vi "main.vi"() -> ()   [LabVIEW 2023]
uses:
  GlobalVariable/SystemMotionLogic.ctl
  Vls/GlobalVariant.vi
  <vilib>/Instr/_visa.llb/VISA Configure Serial Port (Instr).vi
panel:
  in  "Numeric":i32
  in  "StrList":i32[](listbox)
  in  "HexSend":bool
  in  "ClearScreen":bool
  in  "HexDis":bool
  in  "TerminationChar":u8=10 format="%x"
  out "BuffPanel":string
  in  "SendBuffer":string
  in  "BlankButton":bool
  out "IgnoreError":errorcluster
  out "ReadBuffer":string
  in  "Error":errorcluster
  in  "BaudRate":u32=9600
  in  "VISAName":refnum<visa-resource-name>
  in  "Open":bool
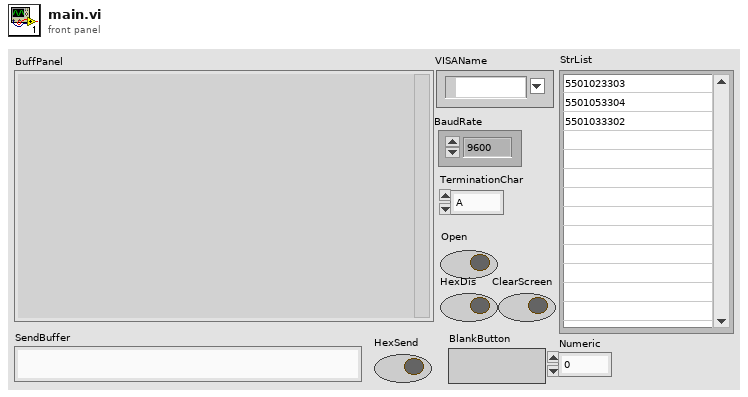
[diagram p1: front panel]
types:
  T1 = typedef "SystemMotionLogic.ctl" = enum16{"VariantInit", "FunctInit", "IdleState"}
  T2 = typedef "LVPoint32TypeDef.ctl" = cluster{"Horizontal":i32, "Vertical":i32}
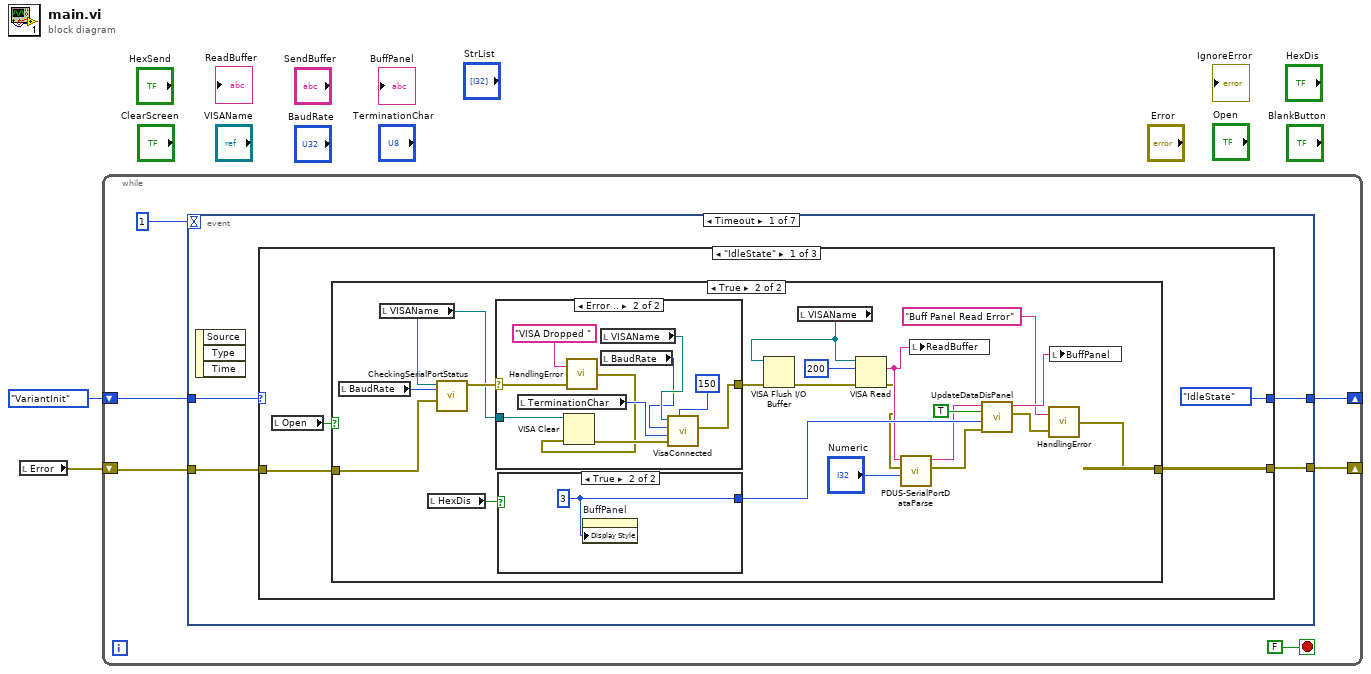
[diagram p0: block diagram]
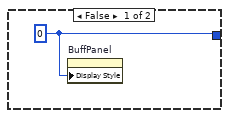
[diagram p4: hidden frame]
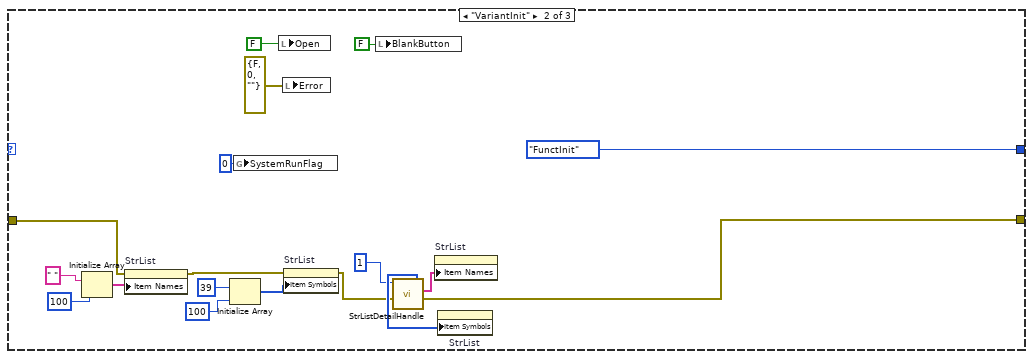
[diagram p5: hidden frame]
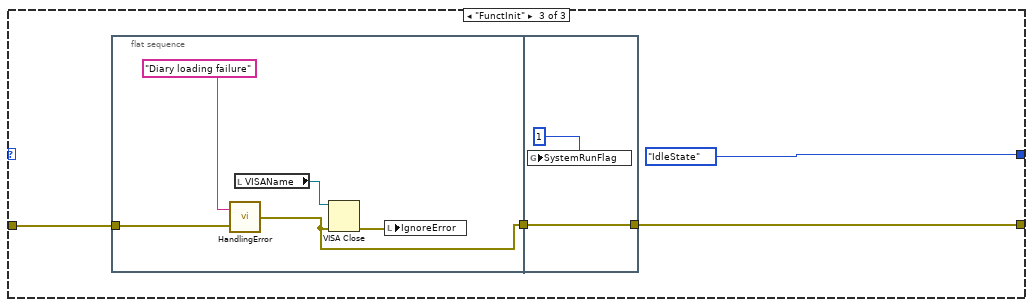
[diagram p6: hidden frame]
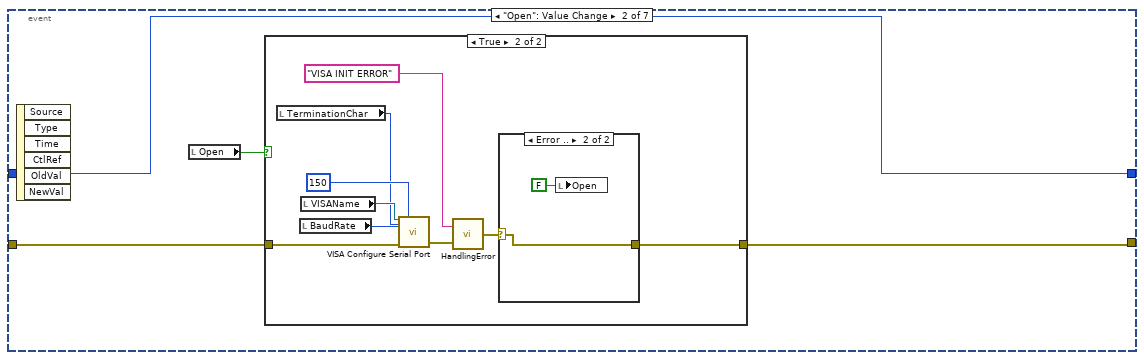
[diagram p7: hidden frame]
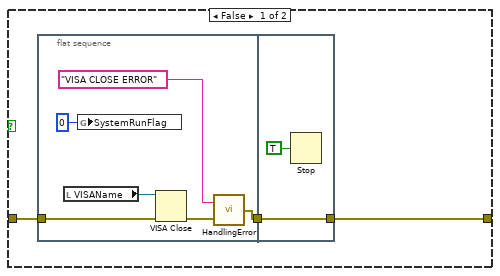
[diagram p8: hidden frame]
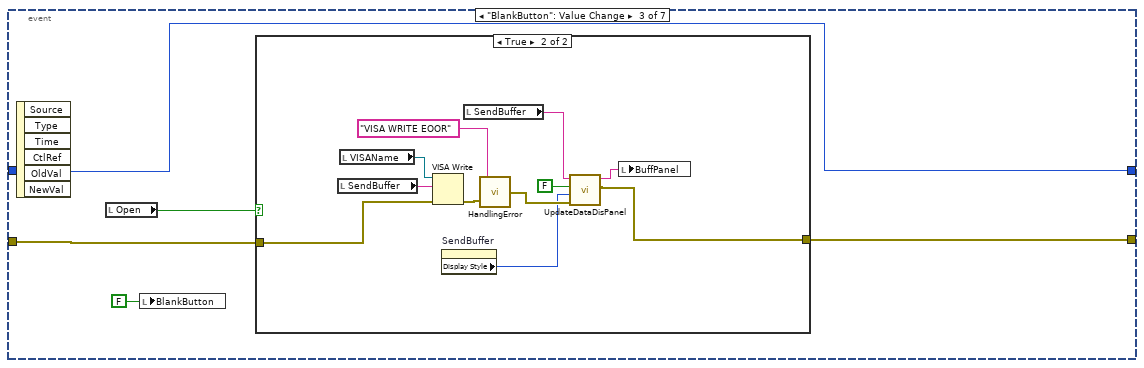
[diagram p10: hidden frame]
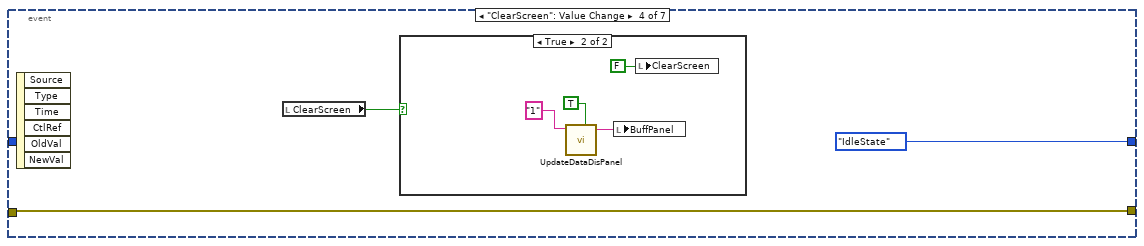
[diagram p12: hidden frame]
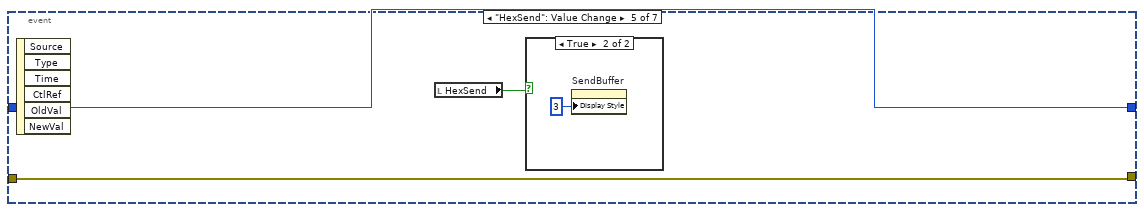
[diagram p14: hidden frame]
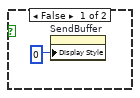
[diagram p15: hidden frame]
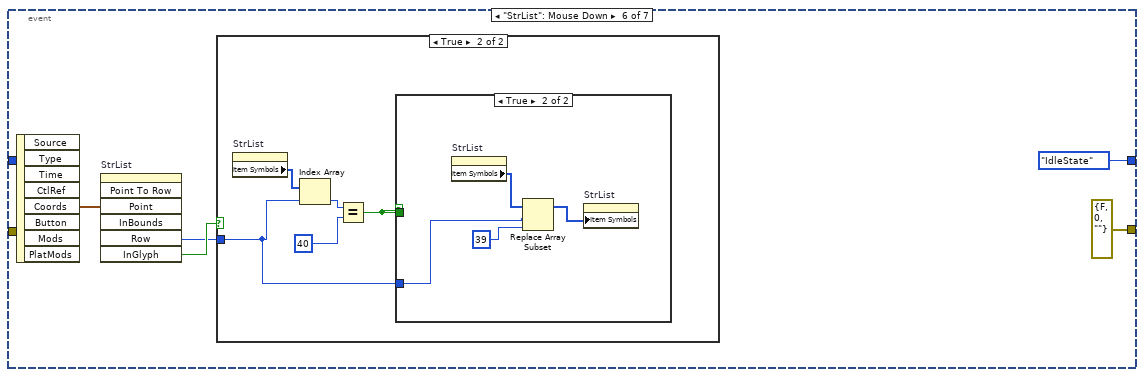
[diagram p16: hidden frame]
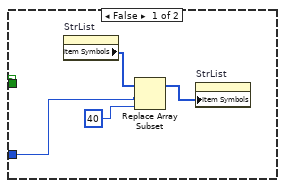
[diagram p18: hidden frame]
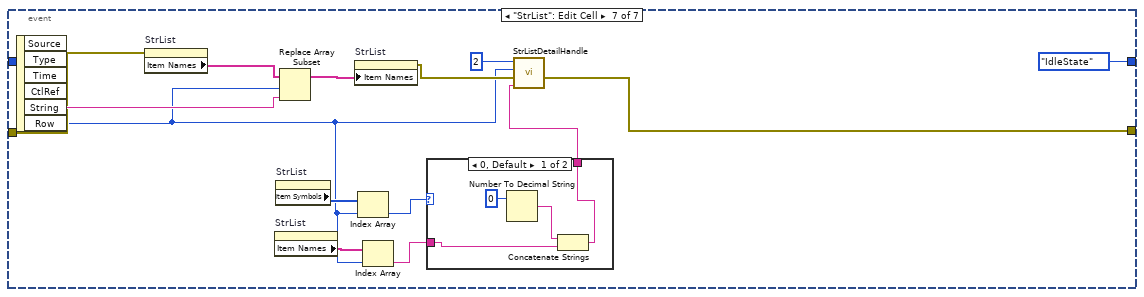
[diagram p19: hidden frame]
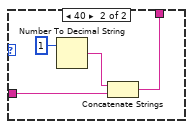
[diagram p20: hidden frame]
diagram:
  n1 = local read "Error"() -> (w2:errorcluster)
  n2 = while {
    shift-right: [w6] -> _
    shift-left: w2 -> [w5]
    shift-right: [w3] -> _
    shift-left: SystemMotionLogic."VariantInit" ("Enum") -> [w4]
    stop <- FALSE stop-if-true
    n3 = event shown="[0] Timeout" {
      selector: _ -> [_ _ _ _ _ _ _]
      dyn-events: _ -> [_ _ _ _ _ _ _]
      timeout: 1 -> [_ _ _ _ _ _ _]
      tunnel: [w11 w82 w109 w125 w132 errorcluster {"status"=FALSE, "code"=0, "source"=""} ("error out") w160] -> w6
      tunnel: w5 -> [w12 w81 w110 w125 w132 _ w163]
      tunnel: w4 -> [w10 w80 w108 _ w131 _ _]
      tunnel: [w9 w80 w108 SystemMotionLogic."IdleState" ("Enum") w131 SystemMotionLogic."IdleState" ("Enum") SystemMotionLogic."IdleState" ("Enum")] -> w3
      event Timeout {
        n4 = event-data() -> ()  [unwired: 1 in, 3 out]
        n5 = case shown="\"IdleState\"" w10 {
          tunnel: w12 -> [w15 w52 w72]
          tunnel: [w14 w51 w71] -> w11
          tunnel: [SystemMotionLogic."IdleState" ("Enum") SystemMotionLogic."FunctInit" ("Enum") SystemMotionLogic."IdleState" ("Enum")] -> w9
          frame "IdleState" {
            n6 = local read "Open"() -> (w16:bool)
            n7 = case shown="True" w16 {
              tunnel: w15 -> [w17 w29]
              tunnel: [w17 w31] -> w14
              frame False {
              }
              frame True {
                n8 = local read "BaudRate"() -> (w23:u32)
                n9 = local read "VISAName"() -> (w27:refnum<visa-resource-name>)
                n10 = local read "HexDis"() -> (w36:bool)
                n11 = call "CheckingSerialPortStatus.vi"("error in"=w29, "Baud"=w23, "VISA  name"=w27) -> ("error output"=w28:errorcluster)  [unwired: 8 in]
                n12 = case shown="Error .." w28 {
                  selector: w28 -> [w38 w47]
                  tunnel: [w38 w46] -> w25
                  tunnel: w27 -> [_ w41]
                  frame No Error {
                  }
                  frame Error {
                    n13 = local read "TerminationChar"() -> (w43:u8)
                    n14 = call "HandlingError.vi"("error input"=w47, "reminder"="VISA Dropped ") -> ("error output"=w40:errorcluster)
                    n15 = VISA Clear(VISA resource name=w41, error in (no error)=w40) -> (error out=w42:errorcluster)  [unwired: 1 out]
                    n16 = local read "VISAName"() -> (w45:refnum<visa-resource-name>)
                    n17 = local read "BaudRate"() -> (w44:u32)
                    n18 = call "VisaConnected.vi"("timeout"=u32 150, "ErrorIn"=w42, "TerminationChar"=w43, "BaudRate"=w44, "VISAName"=w45) -> ("ErrorOut"=w46:errorcluster)  [unwired: 6 in]
                  }
                }
                n19 = case shown="True" w36 {
                  tunnel: [w49 w50] -> w30
                  frame False {
                    w49 = u32 0 ("Display Style")
                    n20 = property on="BuffPanel" class="Str"("Display Style"=w49) -> ()  [unwired: 2 in, 2 out]
                  }
                  frame True {
                    w50 = u32 3 ("Display Style")
                    n21 = property on="BuffPanel" class="Str"("Display Style"=w50) -> ()  [unwired: 2 in, 2 out]
                  }
                }
                n22 = local read "VISAName"() -> (w24:refnum<visa-resource-name>)
                n23 = VISA Flush I/O Buffer(VISA resource name=w24, error in (no error)=w25) -> (error out=w26:errorcluster)  [unwired: 1 in, 1 out]
                n24 = VISA Read(VISA resource name=w24, byte count=u32 200, error in (no error)=w26) -> (read buffer=w22:string, error out=w21:errorcluster)  [unwired: 2 out]
                n25 = call "PDUS-SerialPortDataParse.vi"("Numeric"="Numeric", "ErrorIntput"=w21, "InputStr"=w22) -> ("ErrorOutput"=w20:errorcluster, "OutputStr"=w19:string)  [unwired: 7 in]
                n26 = local write "ReadBuffer"(w22) -> ()
                n27 = call "UpdateDataDisPanel.vi"("Input String"=w19, "send/read"=TRUE, "Display Style"=w30, "error in"=w20) -> ("Output String"=w34:string, "error out"=w35:errorcluster)  [unwired: 4 in]
                n28 = call "HandlingError.vi"("error input"=w35, "reminder"="Buff Panel Read Error") -> ("error output"=w31:errorcluster)
                n29 = local write "BuffPanel"(w34) -> ()
              }
            }
          }
          frame "VariantInit" {
            n30 = Initialize Array(" ", 100 ("dimension size")) -> (w61:string[])
            n31 = property on="StrList" class="LstBox (strict)"(error in=w52, "Item Names"=w61) -> (error out=w57:errorcluster)  [unwired: 1 in, 1 out]
            n32 = Initialize Array(39, 100 ("dimension size")) -> (w58:i32[])
            n33 = global write "GlobalVariant.vi" "SystemRunFlag"(u16 0 ("SystemRunFlag")) -> ()
            n34 = local write "Open"(FALSE ("Stop")) -> ()
            n35 = local write "Error"(errorcluster {"status"=FALSE, "code"=0, "source"=""} ("error")) -> ()
            n36 = property on="StrList" class="LstBox (strict)"(error in=w57, "Item Symbols"=w58) -> (error out=w54:errorcluster)  [unwired: 1 in, 1 out]
            n37 = local write "BlankButton"(FALSE ("Blank Button")) -> ()
            n38 = call "StrListDetailHandle.vi"("ErrorIn"=w54, "MethodChoose"=1) -> ("ErrorOut"=w51:errorcluster, "ItemNames"=w56:string[], "ItemSymbols"=w55:i32[])  [unwired: 3 in]
            n39 = property on="StrList" class="LstBox (strict)"("Item Names"=w56) -> ()  [unwired: 2 in, 2 out]
            n40 = property on="StrList" class="LstBox (strict)"("Item Symbols"=w55) -> ()  [unwired: 2 in, 2 out]
          }
          frame "FunctInit" {
            n41 = flat-sequence {
              tunnel: w72 -> [w77]
              tunnel: [w74] -> w69
              tunnel: [w79] -> w71
              tunnel: w69 -> [w79]
              frame #0 {
                n42 = call "HandlingError.vi"("error input"=w77, "reminder"="Diary loading failure") -> ("error output"=w74:errorcluster)
                n43 = local read "VISAName"() -> (w75:refnum<visa-resource-name>)
                n44 = VISA Close(VISA resource name=w75, error in (no error)=w74) -> (error out=w73:errorcluster)
                n45 = local write "IgnoreError"(w73) -> ()
              }
              frame #1 {
                n46 = global write "GlobalVariant.vi" "SystemRunFlag"(1) -> ()
              }
            }
          }
        }
      }
      event "Open": Value Change {
        n47 = event-data() -> ()  [unwired: 1 in, 6 out]
        n48 = local read "Open"() -> (w83:bool)
        n49 = case shown="True" w83 {
          tunnel: [w85 w96] -> w82
          tunnel: w81 -> [w86 w100]
          frame False {
            n50 = flat-sequence {
              tunnel: w86 -> [w91]
              tunnel: [w89] -> w84
              tunnel: [w94] -> w85
              tunnel: w84 -> [w94]
              frame #0 {
                n51 = local read "VISAName"() -> (w92:refnum<visa-resource-name>)
                n52 = global write "GlobalVariant.vi" "SystemRunFlag"(u16 0 ("SystemRunFlag")) -> ()
                n53 = VISA Close(VISA resource name=w92, error in (no error)=w91) -> (error out=w90:errorcluster)
                n54 = call "HandlingError.vi"("error input"=w90, "reminder"="VISA CLOSE ERROR") -> ("error output"=w89:errorcluster)
              }
              frame #1 {
                n55 = Stop(stop? (T)=TRUE) -> ()
              }
            }
          }
          frame True {
            n56 = local read "TerminationChar"() -> (w95:u8)
            n57 = local read "BaudRate"() -> (w102:u32)
            n58 = local read "VISAName"() -> (w103:refnum<visa-resource-name>)
            n59 = call-poly "VISA Configure Serial Port"("VISA resource name"=w103, "timeout (10sec)"=u32 150, "termination char\n(0xA = '\\n' = LF)"=w95, "baud rate (9600)"=w102, "error in (no error)"=w100) -> ("error out"=w99:errorcluster)  [unwired: 9 in, 1 out]
            n60 = call "HandlingError.vi"("error input"=w99, "reminder"="VISA INIT ERROR") -> ("error output"=w97:errorcluster)
            n61 = case shown="Error .." w97 {
              selector: w97 -> [w104 w105]
              tunnel: [w104 w105] -> w96
              frame No Error {
              }
              frame Error {
                n62 = local write "Open"(FALSE ("OPEN")) -> ()
              }
            }
          }
        }
      }
      event "BlankButton": Value Change {
        n63 = event-data() -> ()  [unwired: 1 in, 6 out]
        n64 = local read "Open"() -> (w111:bool)
        n65 = local write "BlankButton"(FALSE ("OPEN")) -> ()
        n66 = case shown="True" w111 {
          tunnel: w110 -> [w112 w113]
          tunnel: [w112 w118] -> w109
          frame False {
          }
          frame True {
            n67 = local read "SendBuffer"() -> (w122:string)
            n68 = local read "VISAName"() -> (w123:refnum<visa-resource-name>)
            n69 = VISA Write(VISA resource name=w123, write buffer=w122, error in (no error)=w113) -> (error out=w121:errorcluster)  [unwired: 2 out]
            n70 = property on="SendBuffer" class="Str"() -> ("Display Style"=w114:u32)  [unwired: 2 in, 2 out]
            n71 = local read "SendBuffer"() -> (w115:string)
            n72 = call "HandlingError.vi"("error input"=w121, "reminder"="VISA WRITE EOOR") -> ("error output"=w119:errorcluster)
            n73 = call "UpdateDataDisPanel.vi"("Input String"=w115, "send/read"=FALSE, "Display Style"=w114, "error in"=w119) -> ("Output String"=w117:string, "error out"=w118:errorcluster)  [unwired: 4 in]
            n74 = local write "BuffPanel"(w117) -> ()
          }
        }
      }
      event "ClearScreen": Value Change {
        n75 = event-data() -> ()  [unwired: 1 in, 6 out]
        n76 = local read "ClearScreen"() -> (w126:bool)
        n77 = case shown="True" w126 {
          frame False {
          }
          frame True {
            n78 = call "UpdateDataDisPanel.vi"("Input String"="1", "Clear Screen"=TRUE) -> ("Output String"=w127:string)  [unwired: 6 in, 1 out]
            n79 = local write "BuffPanel"(w127) -> ()
            n80 = local write "ClearScreen"(FALSE ("Clear Screen")) -> ()
          }
        }
      }
      event "HexSend": Value Change {
        n81 = event-data() -> ()  [unwired: 1 in, 6 out]
        n82 = local read "HexSend"() -> (w133:bool)
        n83 = case shown="True" w133 {
          frame False {
            n84 = property on="SendBuffer" class="Str"("Display Style"=u32 0) -> ()  [unwired: 2 in, 2 out]
          }
          frame True {
            n85 = property on="SendBuffer" class="Str"("Display Style"=u32 3) -> ()  [unwired: 2 in, 2 out]
          }
        }
      }
      event "StrList": Mouse Down {
        n86 = event-data() -> ("Coords"=w138:T2)  [unwired: 1 in, 7 out]
        n87 = invoke on="StrList" class="LstBox (strict)" method="Point To Row"("Point"=w138) -> ("Row"=w136:i32, "InGlyph"=w137:bool)  [unwired: 6 in, 5 out]
        n88 = case shown="True" w137 {
          tunnel: w136 -> [_ w142]
          frame False {
          }
          frame True {
            n89 = property on="StrList" class="LstBox (strict)"() -> ("Item Symbols"=w143:i32[])  [unwired: 2 in, 2 out]
            n90 = Index Array(array=w143, index=w142) -> (element=w145:i32)
            n91 = Equal?(x=w145, y=40) -> (x = y?=w141:bool)
            n92 = case shown="True" w141 {
              tunnel: w141 -> [_ _]
              tunnel: w142 -> [w146 w151]
              frame False {
                n93 = property on="StrList" class="LstBox (strict)"() -> ("Item Symbols"=w149:i32[])  [unwired: 2 in, 2 out]
                n94 = Replace Array Subset(array=w149, new element=40 ("new element/subarray"), index=w146) -> (w148:i32[])
                n95 = property on="StrList" class="LstBox (strict)"("Item Symbols"=w148) -> ()  [unwired: 2 in, 2 out]
              }
              frame True {
                n96 = property on="StrList" class="LstBox (strict)"() -> ("Item Symbols"=w153:i32[])  [unwired: 2 in, 2 out]
                n97 = Replace Array Subset(array=w153, new element=39 ("new element/subarray"), index=w151) -> (w150:i32[])
                n98 = property on="StrList" class="LstBox (strict)"("Item Symbols"=w150) -> ()  [unwired: 2 in, 2 out]
              }
            }
          }
        }
      }
      event "StrList": Edit Cell {
        n99 = event-data() -> ("String"=w166:string, "Row"=w156:i32)  [unwired: 1 in, 4 out]
        n100 = property on="StrList" class="LstBox (strict)"(error in=w163) -> ("Item Names"=w167:string[])  [unwired: 1 in, 2 out]
        n101 = property on="StrList" class="LstBox (strict)"() -> ("Item Names"=w157:string[])  [unwired: 2 in, 2 out]
        n102 = property on="StrList" class="LstBox (strict)"() -> ("Item Symbols"=w159:i32[])  [unwired: 2 in, 2 out]
        n103 = Replace Array Subset(array=w167, new element=w166, index=w156) -> (w165:string[])
        n104 = property on="StrList" class="LstBox (strict)"("Item Names"=w165) -> (error out=w161:errorcluster)  [unwired: 2 in, 1 out]
        n105 = Index Array(array=w159, index=w156) -> (element=w158:i32)
        n106 = Index Array(array=w157, index=w156) -> (element=w155:string)
        n107 = case shown="0, Default" w158 {
          tunnel: w155 -> [w169 w173]
          tunnel: [w168 w172] -> w154
          frame 0, Default {
            n108 = Number To Decimal String(number=0) -> (decimal integer string=w171:string)  [unwired: 1 in]
            n109 = Concatenate Strings(w171, w169) -> (w168:string)
          }
          frame 40 {
            n110 = Number To Decimal String(number=1) -> (decimal integer string=w174:string)  [unwired: 1 in]
            n111 = Concatenate Strings(w174, w173) -> (w172:string)
          }
        }
        n112 = call "StrListDetailHandle.vi"("Text"=w154, "ErrorIn"=w161, "StrIndex"=w156, "MethodChoose"=2) -> ("ErrorOut"=w160:errorcluster)  [unwired: 1 in, 2 out]
      }
    }
  }
